vi "Set Voltage and Current.vi"(0 "Generic Instrument in":refnum<class "Generic Instrument.lvclass">, 5 "Card #":u8, 7 "Voltage enum number":u16, 9 "Current enum number":u16, 11 "error in (no error)":errorcluster) -> (4 "Generic Instrument out":refnum<class "Generic Instrument.lvclass">, 15 "error out":errorcluster)   [LabVIEW 2016, in "Generic Instrument.lvlib" / "Generic Instrument.lvclass"]
uses:
  Generic Instrument.lvclass
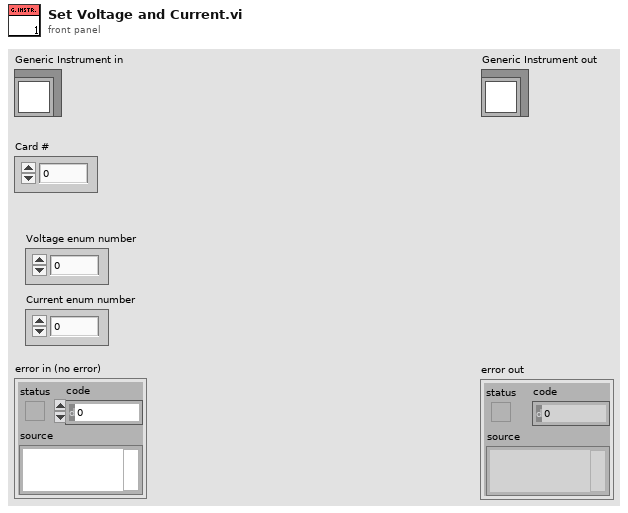
[diagram p1: front panel]
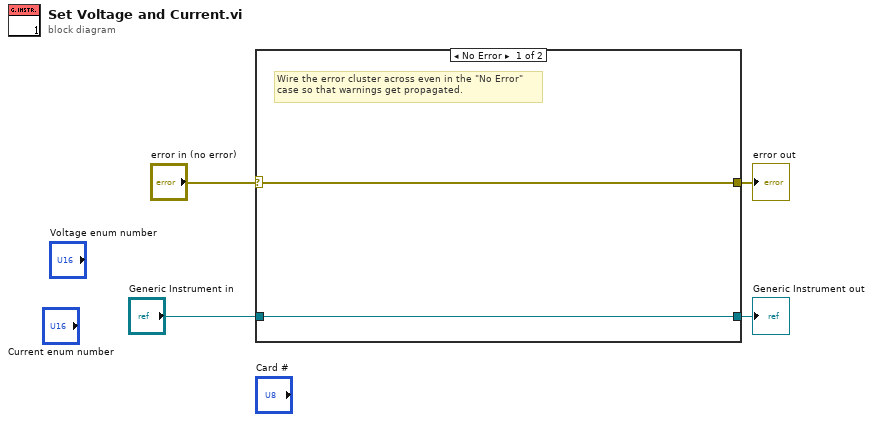
[diagram p0: block diagram]
diagram:
  n1 = case shown="No Error" "error in (no error)" {
    selector: "error in (no error)" -> [w5 w8]
    tunnel: [w5 w8] -> w3
    tunnel: [w6 w7] -> w1
    tunnel: "Generic Instrument in" -> [w6 w7]
    frame No Error {
      # "Wire the error cluster across even in the \"No Error\"\ncase so that warnings get propagated."
    }
    frame Error {
    }
  }
  "error out" <- w3
  "Generic Instrument out" <- w1
